vi "array_test.vi"() -> ()   [LabVIEW 2014]
panel:
  out "deleted portion":cluster{i32, string}
  out "array w/ subset deleted":cluster{i32, string}[](array[cluster])
  out "sorted array":cluster{i32, string}[](array[cluster])
  out "Array":cluster{i32, string}[](array[cluster])=[{3, "trzy"}, {0, "zero"}, {11, "jedenaście"}]
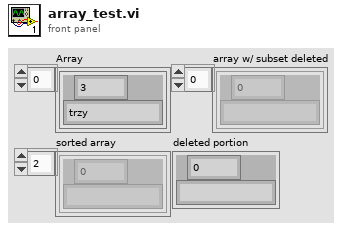
[diagram p1: front panel]
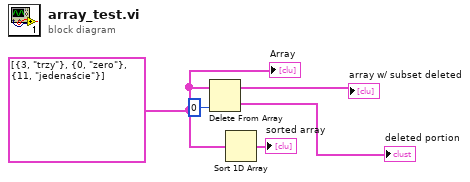
[diagram p0: block diagram]
diagram:
  w4 = cluster{i32, string}[] [{3, "trzy"}, {0, "zero"}, {11, "jedenaście"}]
  n1 = Delete From Array(array=w4, index=0) -> (deleted portion=→"deleted portion":cluster{i32, string}, array with subset deleted=→"array w/ subset deleted":cluster{i32, string}[])  [unwired: 1 in]
  n2 = Sort 1D Array(array=w4) -> (sorted array=→"sorted array":cluster{i32, string}[])
  "Array" <- w4
